vi "DotNetFGV.vi"(8 "Error In":errorcluster, 10 "Operation (Read)":enum16{"Read", "Write"}(ring), 11 "reference in":refnum<k24>) -> (0 "Error Out":errorcluster, 3 "reference out":refnum<k24>)   [LabVIEW 2020]
uses:
  C:/Users/MarcuLab/Documents/GitHub/NetDeconForLV/Source/DotNETAssembly/output/build/LaguerreDeConNative.dll
  Documents/GitHub/NetDeconForLV/Source/DotNETAssembly/output/build/LaguerreDeConNative.dll
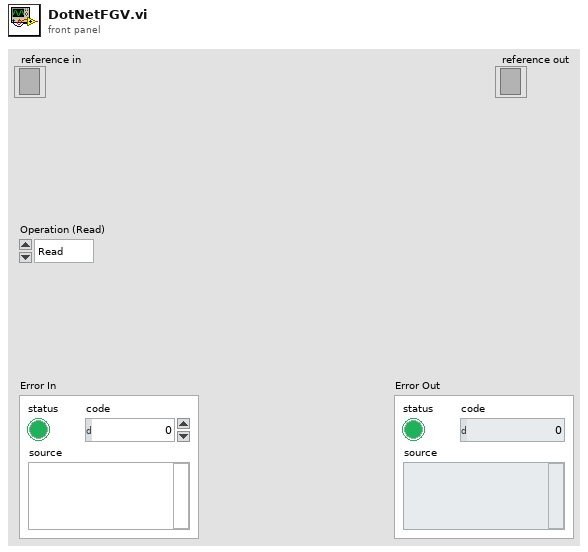
[diagram p1: front panel]
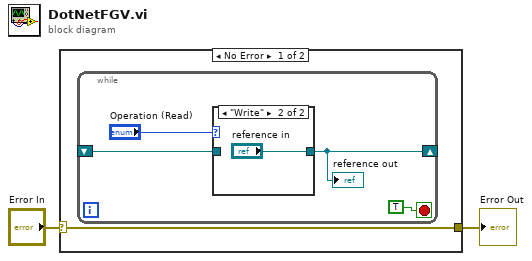
[diagram p0: block diagram]
diagram:
  n1 = case shown="No Error" "Error In" {
    selector: "Error In" -> [w3 w10]
    tunnel: [w3 w10] -> w1
    frame No Error {
      n2 = while {
        shift-right: [w5] -> _
        shift-left: _ -> [w4]
        stop <- TRUE stop-if-true
        n3 = case shown="\"Write\"" "Operation (Read)" {
          tunnel: [w8 "reference in"] -> w5
          tunnel: w4 -> [w8 _]
          frame "Read", Default {
          }
          frame "Write" {
          }
        }
        "reference out" <- w5
      }
    }
    frame Error {
    }
  }
  "Error Out" <- w1
